vi "Execute Turn.vi"(7 "Player Color":T1, 8 "error in":errorcluster, 9 "Possible Moves":bool[][](array[boolean]), 10 "Board":T3[][](array[typedef]), 11 "Human in":refnum<class "Human.lvclass">) -> (0 "error out":errorcluster, 2 "Choice Coordinates":T2, 3 "Human out":refnum<class "Human.lvclass">)   [LabVIEW 2020, in "Human.lvclass"]
uses:
  Human.lvclass
  Space Ring.ctl
  Space Coordinates.ctl
  Turn Enum.ctl
  Human.lvclass/Human.ctl
  Reversi.lvclass
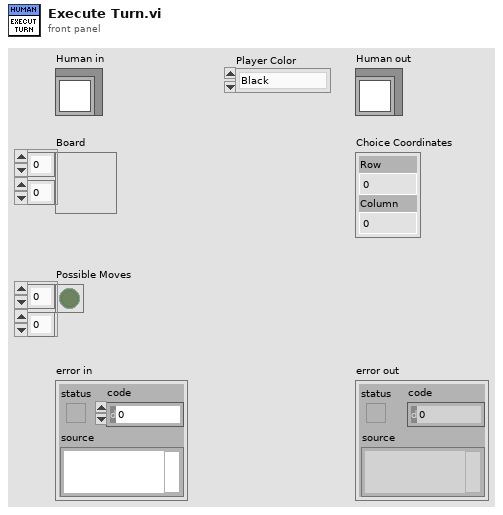
[diagram p1: front panel]
types:
  T1 = typedef "Reversi.lvlib/Reversi.lvclass/Turn Enum.ctl" = enum16{"Black", "White"}
  T2 = typedef "Reversi.lvlib/Reversi.lvclass/Space Coordinates.ctl" = cluster{"Row":i32, "Column":i32}
  T3 = typedef "Reversi.lvlib/Reversi.lvclass/Space Ring.ctl" = u16
  T4 = typedef "LVPoint32TypeDef.ctl" = cluster{"Horizontal":i32, "Vertical":i32}
  T5 = typedef "LVPositionTypeDef.ctl" = cluster{"Left":i32, "Top":i32}
  T6 = typedef "LVBoundsTypeDef.ctl" = cluster{"Width":u32, "Height":u32}
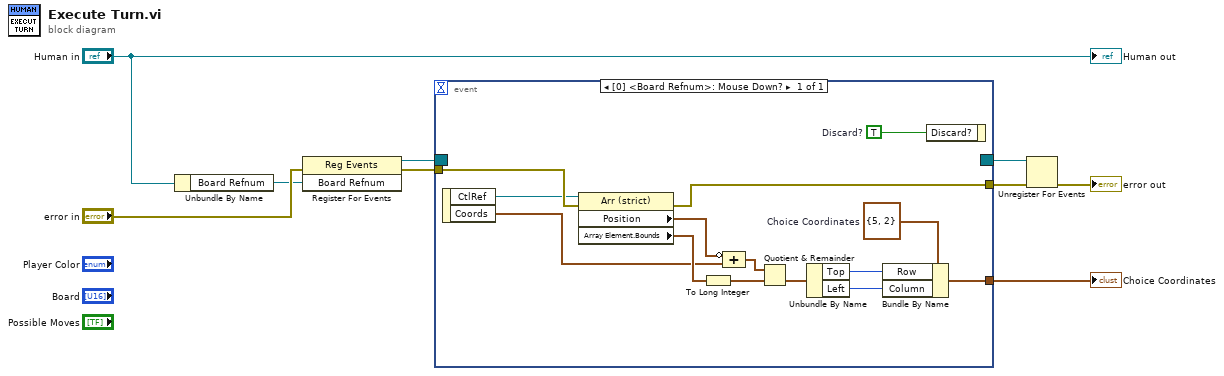
[diagram p0: block diagram]
diagram:
  n1 = Unbundle By Name("Human in") -> ("Board Refnum"=w4:refnum<vi>)
  n2 = register-events(error in="error in", w4) -> (reference out=w3:refnum<event-registration>, error out=w8:errorcluster)  [unwired: 1 in]
  n3 = event shown="[0] <Board Refnum>: Mouse Down?" {
    selector: w3 -> [_]
    dyn-events: [_] -> w1
    timeout: _ -> [_]
    tunnel: w8 -> [w23]
    tunnel: [w13] -> w2
    tunnel: [w22] -> w7
    event Mouse Down? {
      w14 = T2 {"Row"=5, "Column"=2}  # Choice Coordinates
      w21 = TRUE  # Discard?
      n4 = event-data() -> ("CtlRef"=w20:refnum<vi>, "Coords"=w18:T4)  [unwired: 1 in]
      n5 = property class="Arr (strict)"(reference=w20, error in=w23) -> (error out=w22:errorcluster, "Position"=w17:T5, "Array Element.Bounds"=w19:T6)  [unwired: 1 out]
      n6 = To Long Integer(number=w19) -> (32bit integer=w15:cluster{"Width":i32, "Height":i32})
      n7 = Compound Arithmetic op=ADD(invert w17, w18) -> (w16:T5)
      n8 = Quotient & Remainder(x=w16, y=w15) -> (floor(x/y)=w12:T5)  [unwired: 1 out]
      n9 = Unbundle By Name(w12) -> ("Top"=w11:i32, "Left"=w10:i32)
      n10 = Bundle By Name(cluster=w14, "Row"=w11, "Column"=w10) -> (w13:T2)
      n11 = event-data("Discard?"=w21) -> ()  [unwired: 1 in, 1 out]
    }
  }
  "Choice Coordinates" <- w2
  n12 = Unregister For Events(event registration refnum=w1, error in=w7) -> (error out=→"error out":errorcluster)
  "Human out" <- "Human in"
